vi "MPXsetSignal.vi"(2 "Refresh":bool, 3 "Waveform":u16(ring) items=["Sine", "Rectangle", "SRS-Signal"], 4 "Comport in":refnum<visa-resource-name>="COM8") -> (0 "read buffer":string="MS\r\nWaveform changed\r\n\r\nWavetype: Sine\r\nFrequence: 0100 Hz\r\nAmplitude: 250 Vpp\r\nSignal off\r\n\r\nempc>:\n", 1 "Comport out":refnum<visa-resource-name>="COM8")   [LabVIEW 2015]
uses:
  Instance           1 21Saved   MPX setSignal .vi
panel:
  out "Boolean":bool=TRUE
  out "Waveform bkp":u16(ring) items=["Sine", "Rectangle", "SRS-Signal"]
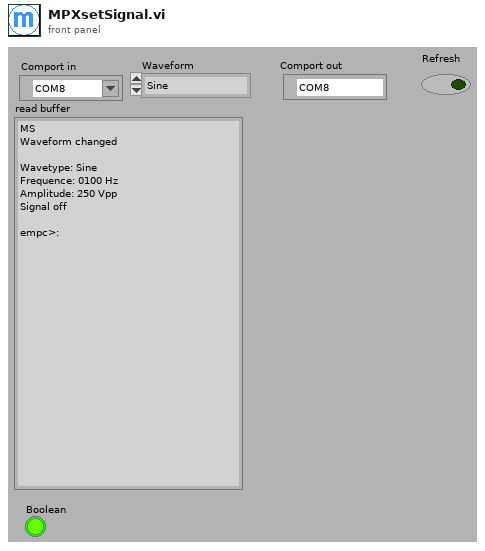
[diagram p1: front panel]
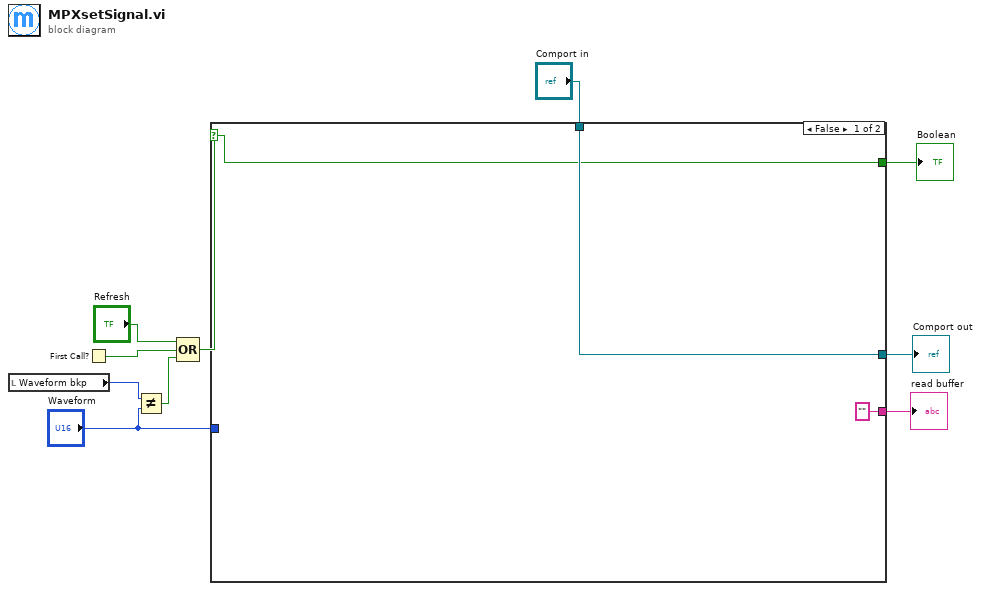
[diagram p0: block diagram]
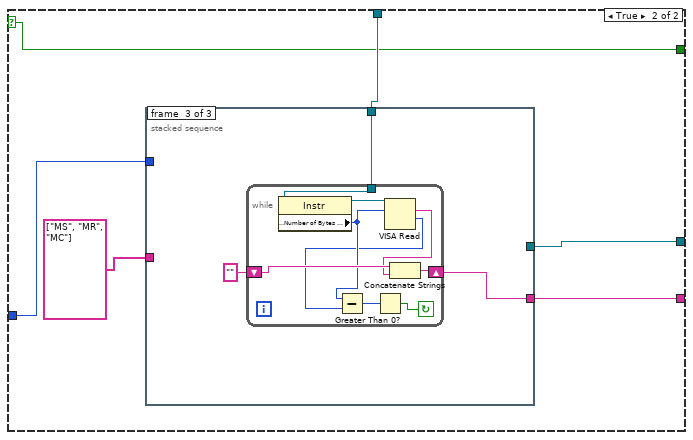
[diagram p2: hidden frame]
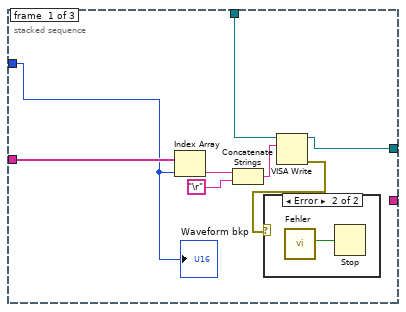
[diagram p3: hidden frame]
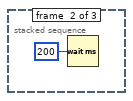
[diagram p5: hidden frame]
diagram:
  n1 = local read "Waveform bkp"() -> (w3:u16)
  n2 = First Call?() -> (First Call?: T/F=w6:bool)
  n3 = Not Equal?(x=w3, y="Waveform") -> (x != y?=w4:bool)
  n4 = Compound Arithmetic op=OR("Refresh", w6, w4) -> (w8:bool)
  n5 = case shown="False" w8 {
    selector: w8 -> [w12 w15]
    tunnel: "Comport in" -> [w13 w18]
    tunnel: [w13 w17] -> w9
    tunnel: "Waveform" -> [_ w16]
    tunnel: [w12 w15] -> w2
    tunnel: ["" w14] -> w1
    frame False {
    }
    frame True {
      n6 = stacked-sequence {
        tunnel: string[] ["MS", "MR", "MC"] -> [w27 _ _]
        tunnel: w18 -> [w23 _ w32]
        tunnel: w16 -> [w21 _ _]
        tunnel: [w22 _ _] -> w17
        tunnel: [_ _ w30] -> w14
        frame #0 {
          n7 = Index Array(array=w27, index=w21) -> (element=w26:string)
          n8 = Concatenate Strings(w26, "\r") -> (w24:string)
          n9 = VISA Write(VISA resource name=w23, write buffer=w24) -> (VISA resource name out=w22:refnum<visa-resource-name>, error out=w20:errorcluster)  [unwired: 1 in, 1 out]
          n10 = case shown="Error" w20 {
            frame No Error {
            }
            frame Error {
              n11 = call "Fehler"() -> ("OK"=w28:bool)  [unwired: 10 in, 1 out]
              n12 = Stop(stop? (T)=w28) -> ()
            }
          }
          "Waveform bkp" <- w21
        }
        frame #1 {
          n13 = Wait (ms)(milliseconds to wait=u32 200) -> ()  [unwired: 1 out]
        }
        frame #2 {
          n14 = while {
            shift-right: [w39] -> w30
            shift-left: "" -> [w40]
            tunnel: w32 -> [w33]
            stop <- w34 continue-if-true
            n15 = property class="Instr"(reference=w33) -> (reference out=w41:refnum<visa-resource-name>, "Serial Settings:Number of Bytes at Serial Port"=w36:u32)  [unwired: 1 in, 1 out]
            n16 = VISA Read(VISA resource name=w41, byte count=w36) -> (read buffer=w38:string, return count=w35:u32)  [unwired: 1 in, 2 out]
            n17 = Subtract(x=w36, y=w35) -> (x-y=w37:u32)
            n18 = Greater Than 0?(x=w37) -> (x > 0?=w34:bool)
            n19 = Concatenate Strings(w40, w38) -> (w39:string)
          }
        }
      }
    }
  }
  "Comport out" <- w9
  "Boolean" <- w2
  "read buffer" <- w1
